vi "Write_Data.vi"(5 "DB #":u16, 6 "wait for reply (T)":bool=TRUE, 7 "寄存器类型":u8(ring)=132 items=["I/O (P)"=128, "Input (I)"=129, "Output (Q)"=130, "Bit Memory (M)"=131, "Data (DB)"=132, "Instance Data (DI)"=133, "Local Data (L)"=134, "Predecessor Local Data (VL)"=135], 8 "error in (no error)":errorcluster, 9 "写入数据":u32, 10 "数据类型":u16(ring) items=["byte", "word", "Dword"], 11 "写入地址":u32=1) -> (0 "error out":errorcluster, 1 "timed out?":bool, 2 "Reply Payload":T1)   [LabVIEW 2020, in "S7.lvlib"]
doc: "_____\nCreated using Delacor QMH Event Scripter 4.1.0.80."
uses:
  S7.lvlib
  Write_Data (Reply Payload)--cluster.ctl
  Write_Data Argument--cluster.ctl
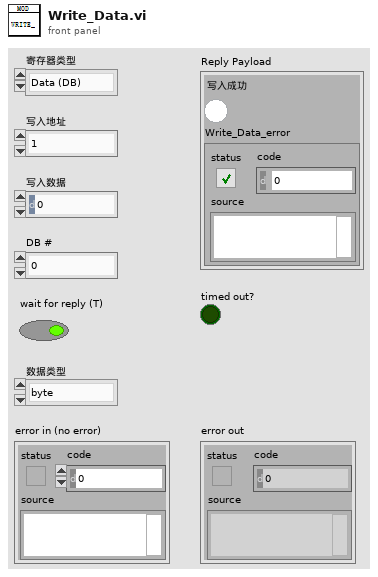
[diagram p1: front panel]
types:
  T1 = typedef "S7.lvlib/Write_Data (Reply Payload)--cluster.ctl" = cluster{"写入成功":bool, "Write_Data_error":errorcluster}
  T2 = typedef "S7.lvlib/Write_Data Argument--cluster.ctl" = cluster{"写入数据":u32, "DB #":u16, "写入地址":u32, "寄存器类型":u8, "数据类型":u16, "Wait Notifier":refnum<notifier>, "wait for reply":bool}
  T3 = typedef "S7.lvlib/Request Events--cluster.ctl" = cluster{"Stop Module":refnum<user-event>, "Show Panel":refnum<user-event>, "Hide Panel":refnum<user-event>, "Get Module Execution Status":refnum<user-event>, "Show Diagram":refnum<user-event>, "S7_Open":refnum<user-event>, "Init S7 Link":refnum<user-event>, "Close S7 Link":refnum<user-event>, "Read_Data":refnum<user-event>, "Write_Data":refnum<user-event>}
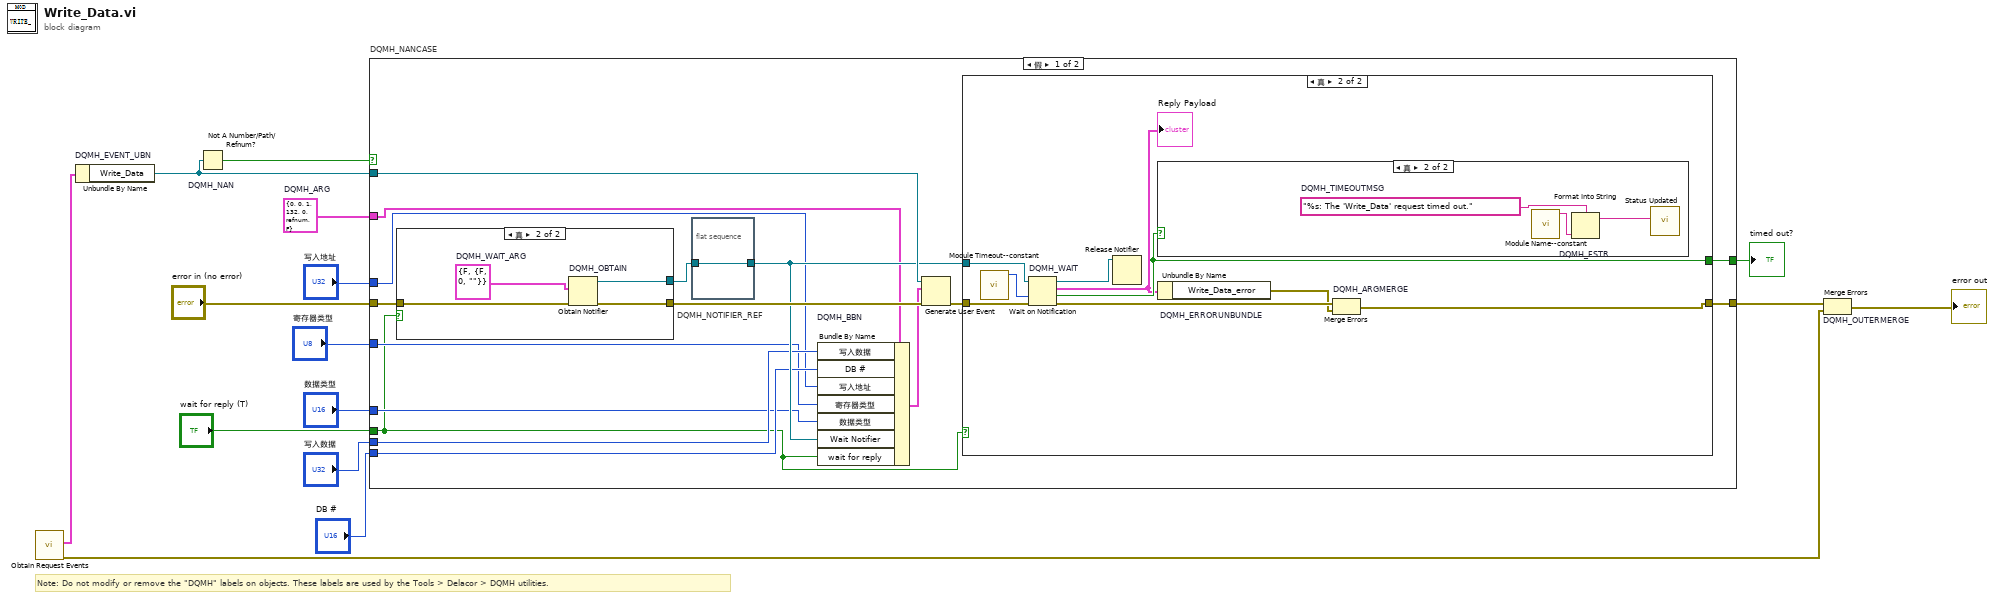
[diagram p0: block diagram]
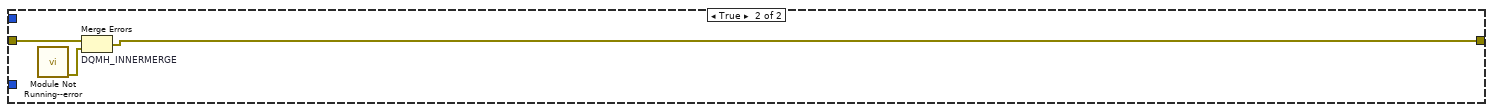
[diagram p5: hidden frame]
diagram:
  w9 = T2 {"写入数据"=0, "DB #"=0, "写入地址"=1, "寄存器类型"=132, "数据类型"=0, "Wait Notifier"=refnum, "wait for reply"=FALSE}  # DQMH_ARG
  # "Note: Do not modify or remove the \"DQMH\" labels on objects. These labels are used by the Tools > Delacor > DQMH utilities."
  n1 = call "Obtain Request Events.vi"() -> ("error out"=w2:errorcluster, "S7 Request Events"=w1:T3)  [unwired: 10 in]
  n2 = Unbundle By Name "DQMH_EVENT_UBN"(w1) -> ("Write_Data"=w13:refnum<user-event>)
  n3 = Not A Number/Path/Refnum? "DQMH_NAN"(number/path/refnum=w13) -> (NaN/Path/Refnum?=w12:bool)
  n4 = case "DQMH_NANCASE" shown="假" w12 {
    tunnel: "error in (no error)" -> [w31 w53]
    tunnel: w13 -> [w29 _]
    tunnel: [w26 w52] -> w10
    tunnel: [w27 _] -> w11
    tunnel: w9 -> [w22 _]
    tunnel: "写入数据" -> [w21 _]
    tunnel: "DB #" -> [w20 _]
    tunnel: "写入地址" -> [w19 _]
    tunnel: "寄存器类型" -> [w18 _]
    tunnel: "数据类型" -> [w17 _]
    tunnel: "wait for reply (T)" -> [w16 _]
    frame False {
      n5 = case shown="真" w16 {
        tunnel: w31 -> [w46 w50]
        tunnel: [w46 w49] -> w28
        tunnel: [_ w47] -> w24
        frame False {
        }
        frame True {
          w48 = T1 {"写入成功"=FALSE, "Write_Data_error"={"status"=FALSE, "code"=0, "source"=""}}  # DQMH_WAIT_ARG
          n6 = Obtain Notifier "DQMH_OBTAIN"(notification data type=w48, error in (no error)=w50) -> (notifier out=w47:refnum<notifier>, error out=w49:errorcluster)  [unwired: 2 in, 1 out]
        }
      }
      n7 = flat-sequence "DQMH_NOTIFIER_REF" {
        tunnel: w24 -> [w32]
        tunnel: [w32] -> w23
        frame #0 {
        }
      }
      n8 = Bundle By Name "DQMH_BBN"(cluster=w22, "写入数据"=w21, "DB #"=w20, "写入地址"=w19, "寄存器类型"=w18, "数据类型"=w17, "Wait Notifier"=w23, "wait for reply"=w16) -> (w25:T2)
      n9 = Generate User Event(user event=w29, event data cluster=w25, error in=w28) -> (error out=w30:errorcluster)  [unwired: 1 in, 1 out]
      n10 = case "条件结构" shown="真" w16 {
        tunnel: w30 -> [w33 w42]
        tunnel: w23 -> [_ w40]
        tunnel: [_ w38] -> w27
        tunnel: [w33 w37] -> w26
        frame False {
        }
        frame True {
          n11 = call "Module Timeout--constant.vi"() -> ("Module Timeout"=w34:i32)  [unwired: 11 in]
          n12 = Wait on Notification "DQMH_WAIT"(notifier=w40, timeout in ms (-1)=w34, error in (no error)=w42) -> (notifier out=w39:refnum<notifier>, notification=w35:T1, timed out?=w38:bool, error out=w41:errorcluster)  [unwired: 1 in]
          "Reply Payload" <- w35
          n13 = Release Notifier ("释放通知器引用")(notifier=w39) -> ()  [unwired: 2 in, 3 out]
          n14 = case "条件结构" shown="真" w38 {
            frame False {
            }
            frame True {
              w45 = "%s: The 'Write_Data' request timed out."  # DQMH_TIMEOUTMSG
              n15 = call "Module Name--constant.vi"() -> ("Module Name"=w44:string)  [unwired: 11 in]
              n16 = Format Into String "DQMH_FSTR"(format string=w45, w44) -> (resulting string=w43:string)  [unwired: 2 in, 1 out]
              n17 = call "Status Updated.vi"("Status"=w43) -> ()  [unwired: 10 in, 1 out]
            }
          }
          n18 = Unbundle By Name "DQMH_ERRORUNBUNDLE"(w35) -> ("Write_Data_error"=w36:errorcluster)
          n19 = Merge Errors "DQMH_ARGMERGE"(w41, w36) -> (w37:errorcluster)
        }
      }
    }
    frame True {
      n20 = call "Module Not Running--error.vi"() -> ("error out"=w51:errorcluster)  [unwired: 11 in]
      n21 = Merge Errors "DQMH_INNERMERGE"(w53, w51) -> (w52:errorcluster)
    }
  }
  "timed out?" <- w11
  n22 = Merge Errors "DQMH_OUTERMERGE"(w10, w2) -> (→"error out":errorcluster)
